vi "Script Msg Input.vi"(8 "error in":errorcluster, 10 "Name Msg IO (Input)":T1) -> (0 "error out":errorcluster)   [LabVIEW 2025, in "_Rescript.lvlib" / "Msg.lvlib" / "Msg.lvclass"]
uses:
  Msg.lvclass
  Terminal Attributes.ctl
  Attributes.ctl
  <vilib>/Utility/traverseref.llb/TRef TravTarget.ctl
  Msg.lvclass/Msg.ctl
  _Rescript.lvlib
  Name Msg IO.ctl
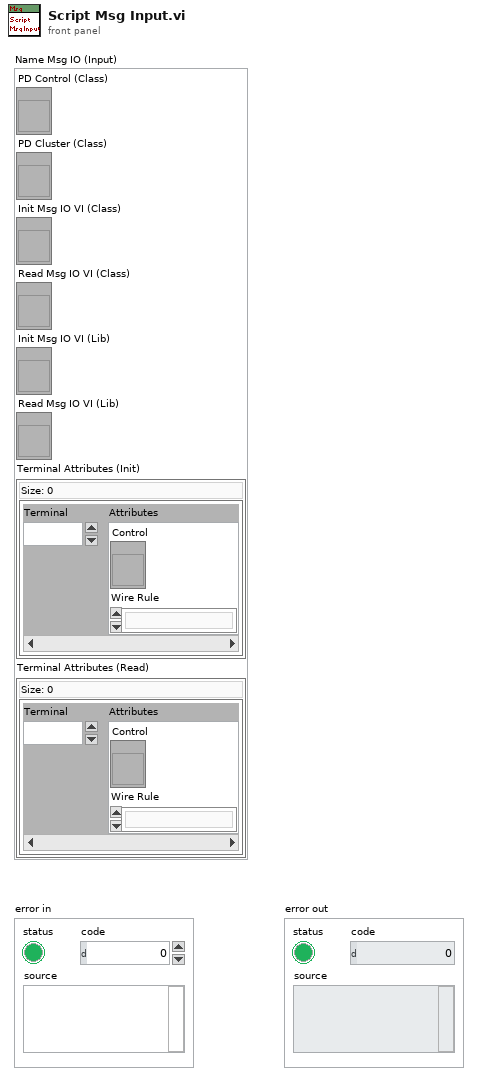
[diagram p1: front panel]
types:
  T1 = typedef "_Rescript.lvlib/Msg.lvlib/Msg.lvclass/Name Msg IO.ctl" = cluster{"PD Control (Class)":refnum<vi>, "PD Cluster (Class)":refnum<vi>, "Init Msg IO VI (Class)":refnum<vi>, "Read Msg IO VI (Class)":refnum<vi>, "Init Msg IO VI (Lib)":refnum<vi>, "Read Msg IO VI (Lib)":refnum<vi>, "Terminal Attributes (Init)":T2, "Terminal Attributes (Read)":T2}
  T2 = typedef "_Rescript.lvlib/Terminal Attributes.ctl" = map{i32, T3}
  T3 = typedef "_Rescript.lvlib/Attributes.ctl" = cluster{"Control":refnum<vi>, "Wire Rule":enum16{"Invalid Wire Rule", "Required", "Recommended", "Optional", "Dynamic Dispatch"}}
  T4 = typedef "TRef TravTarget.ctl" = enum16{"FP", "BD", "Other"}
  T5 = enum16{"Invalid Wire Rule", "Required", "Recommended", "Optional", "Dynamic Dispatch"}
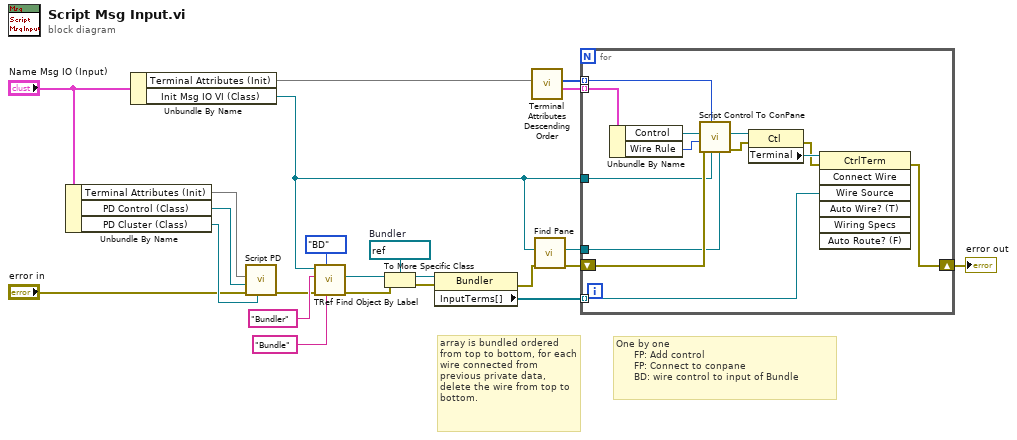
[diagram p0: block diagram]
diagram:
  w19 = refnum<vi> refnum  # Bundler
  # "array is bundled ordered from top to bottom, for each wire connected from previous private data, delete the wire from top to bottom."
  # "One by one\n      FP: Add control\n      FP: Connect to conpane\n      BD: wire control to input of Bundle"
  n1 = Unbundle By Name("Name Msg IO (Input)") -> ("Terminal Attributes (Init)"=w4:T2, "PD Control (Class)"=w5:refnum<vi>, "PD Cluster (Class)"=w6:refnum<vi>)
  n2 = Unbundle By Name("Name Msg IO (Input)") -> ("Terminal Attributes (Init)"=w8:T2, "Init Msg IO VI (Class)"=w7:refnum<vi>)
  n3 = call "Script PD.vi"("PD Cluster"=w6, "error in"="error in", "PD Control"=w5, "Terminal Attributes"=w4) -> ("error out"=w2:errorcluster)  [unwired: 7 in]
  n4 = call <vilib>:"TRef Find Object By Label.vi"("Label"="Bundle", "Traverse Target"=TRef_TravTarget."BD", "error in (no error)"=w2, "Class Name"="Bundler", "VI Ref"=w7) -> ("error out"=w23:errorcluster, "Found Obj Ref"=w22:refnum<vi>)  [unwired: 3 in, 2 out]
  n5 = To More Specific Class(target class=w19, reference=w22, error in=w23) -> (specific class reference=w18:refnum<vi>, error out=w17:errorcluster)
  n6 = property class="Bundler"(reference=w18, error in=w17) -> (error out=w12:errorcluster, "InputTerms[]"=w14:refnum<vi>[])  [unwired: 1 out]
  n7 = call "Terminal Attributes Descending Order.vi"("Terminal Attributes"=w8) -> ("Attributes Descending Order"=w9:T3[], "Terminal Descending Order"=w10:i32[])  [unwired: 9 in]
  n8 = call "Find Pane.vi"("error in"=w12, "VI Ref"=w7) -> ("error out"=w11:errorcluster, "Pane Ref"=w13:refnum<vi>)  [unwired: 8 in]
  n9 = for {
    tunnel: w10 -> [w25] mode=indexing
    tunnel: w13 -> [w29]
    tunnel: w7 -> [w28]
    tunnel: w14 -> [w35] mode=indexing
    shift-right: [w33] -> w15
    shift-left: w11 -> [w30]
    tunnel: w9 -> [w24] mode=indexing
    n10 = Unbundle By Name(w24) -> ("Control"=w27:refnum<vi>, "Wire Rule"=w26:T5)
    n11 = call "Script Control To ConPane.vi"("Pane"=w29, "VI"=w28, "Terminal"=w25, "error in"=w30, "Wire Rule"=w26, "Control To Duplicate"=w27) -> ("error out"=w31:errorcluster, "Duplicated Control"=w32:refnum<vi>)  [unwired: 4 in]
    n12 = property class="Ctl"(reference=w32, error in=w31) -> (error out=w34:errorcluster, "Terminal"=w36:refnum<vi>)  [unwired: 1 out]
    n13 = invoke class="CtrlTerm" method="Connect Wire"(reference=w36, error in=w34, "Wire Source"=w35) -> (error out=w33:errorcluster)  [unwired: 4 in, 6 out]
  }
  "error out" <- w15
